vi "Main.vi"() -> ()   [LabVIEW 2021]
uses:
  Controls/Tab Control.ctl
  Controls/case control.ctl
  Controls/status_amc_entries.ctl
  Controls/assign_amc_status.ctl
  Controls/Enum.ctl
  Controls/MySQL Credential Control.ctl
panel:
  in  "error in (no error) 2":errorcluster
  in  "error in (no error)":errorcluster
  in  "Tab Control":T1
  in  "Password":string
  in  "Username":string
  in  "Login Button":bool
  in  "Role  2":T2
  in  "Assign AMC":bool
  in  "Manage Clients":bool
  in  "Report Button":bool
  in  "ADD/EDIT AMC":bool
  in  "ADD USER":bool
  in  "View All AMC":bool
  in  "Log out":bool
  in  "login Back 1":bool
  in  "Log Service Visit":bool
  in  "View Assigned AMC":bool
  in  "Update AMC":bool
  in  "login Back  2":bool
  in  "View Clients":bool
  in  "View Assign AMC":bool
  in  "View AMC":bool
  in  "Save":bool
  in  "Back":bool
  in  "Role":enum16{"admin", "engineer", "user"}(ring)
  in  "Add Username":string
  in  "Add Password":string
  in  "Delete":bool
  in  "Back Button 2":bool
  in  "User Assigned":string
  in  "Maintenance Cycle":enum16{"Quaterly", "Half Yearly", "Yearly"}(ring)
  in  "AMC Status":T3
  in  "Expiry Date":timestamp format="%<%Y/%m/%d>T"
  in  "Purchase Date":timestamp format="%<%Y/%m/%d>T"
  in  "Vendor":string
  in  "Machine":string
  in  "ADD AMC":bool
  in  "Refresh Button":bool
  in  "Back Button":bool
  out "data":string[][](table)
  in  "Back Button 4":bool
  in  "Assign":bool
  in  "Remarks":string
  in  "Status":T4
  in  "vendor":string
  in  "maintenance_cycle":string
  in  "machine_name":string
  in  "Location":string
  in  "assigned_engineer_id":dbl
  in  "engineer_remarks":string
  out "Table 3":string[][](table)
  in  "Back Button 3":bool
  in  "Back Button 5":bool
  out "Table 2":string[][](table)
  in  "Back Button 6":bool
  in  "Upload Button":bool
  in  "id 3":dbl
  in  "engineer_remarks 3":string
  in  "Back Button 7":bool
  in  "User Back Button":bool
  out "data 3":string[][](table)
  in  "User Back Button 2":bool
  out "Table":string[][](table)
  in  "User Back Button 1":bool
  out "Table 5":string[][](table)
  out "error out":errorcluster
  # "AMC TRACKER"
  # "Admin Dashboard"
  # "Engineer Dashboard"
  # "Status"
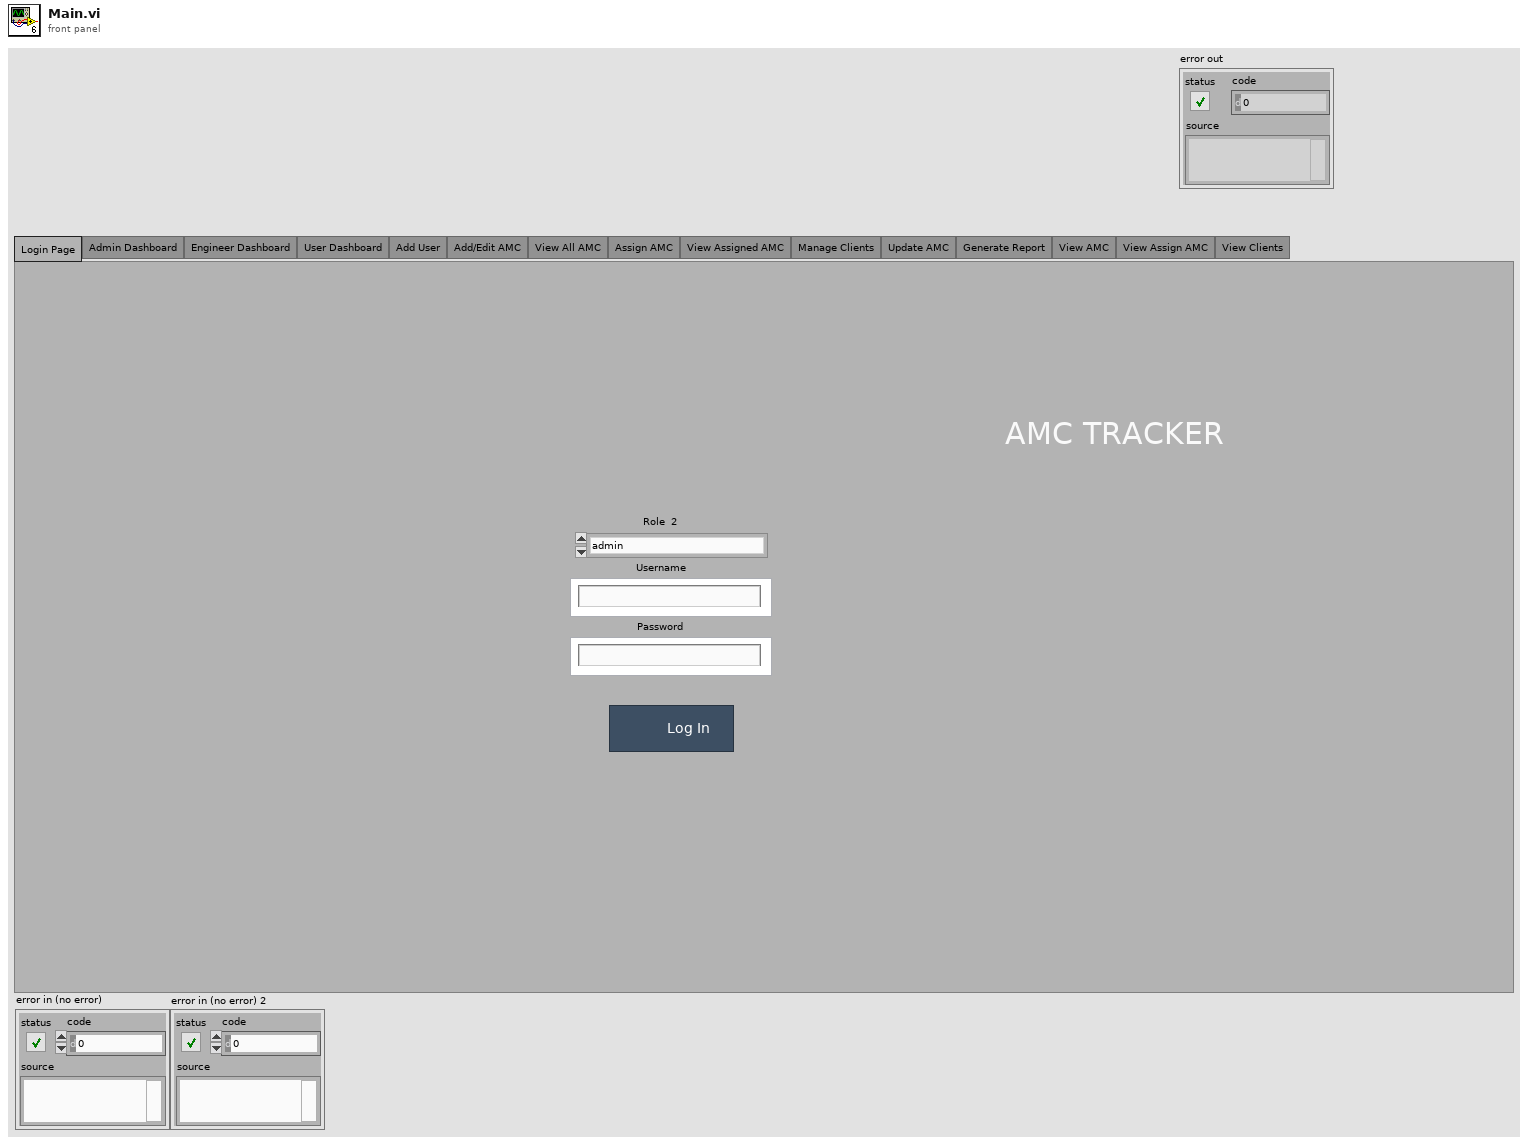
[diagram p1: front panel]
types:
  T1 = typedef "Tab Control.ctl" = enum32{"Login Page", "Admin Dashboard", "Engineer Dashboard", "User Dashboard", "Add User", "Add/Edit AMC", "View All AMC", "Assign AMC", "View Assigned AMC", "Manage Clients", "Update AMC", "Generate Report", "View AMC", "View Assign AMC", "View Clients"}
  T2 = typedef "case control.ctl" = enum16{"admin", "engineer", "user"}
  T3 = typedef "status_amc_entries.ctl" = enum16{"Active", "Expired"}
  T4 = typedef "assign_amc_status.ctl" = enum16{"Active", "Completed", "Pending"}
  T5 = typedef "Enum.ctl" = enum16{"init", "Execute Query", "Close"}
  T6 = typedef "MySQL Credential Control.ctl" = cluster{"Server":string, " User ID":string, "Password":string}
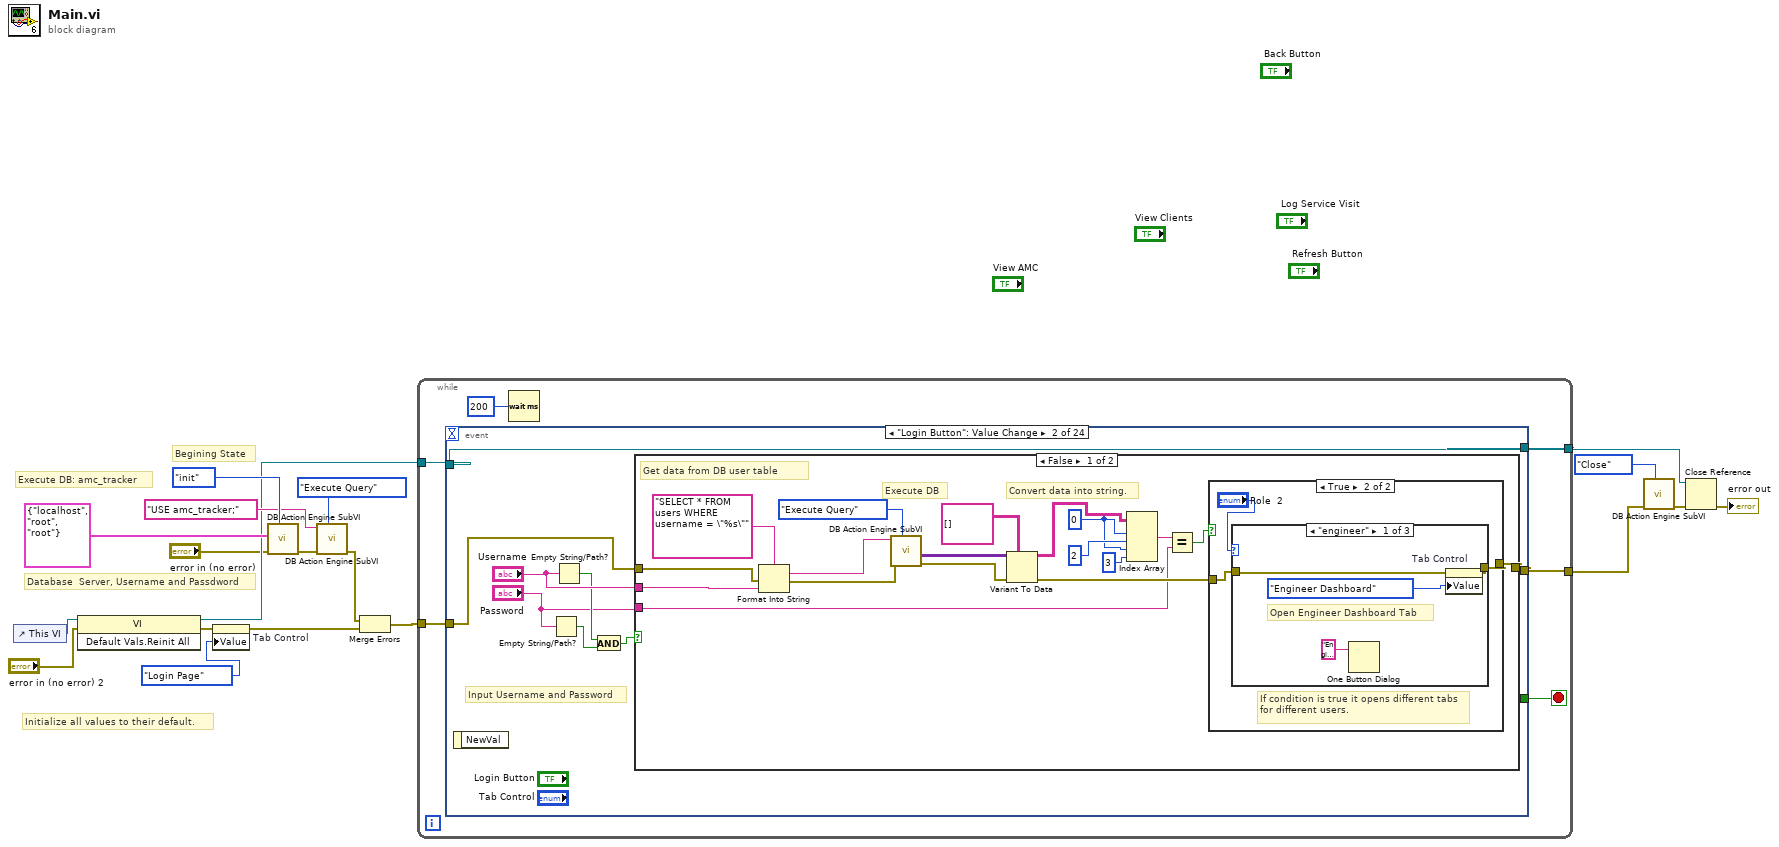
[diagram p0: block diagram]
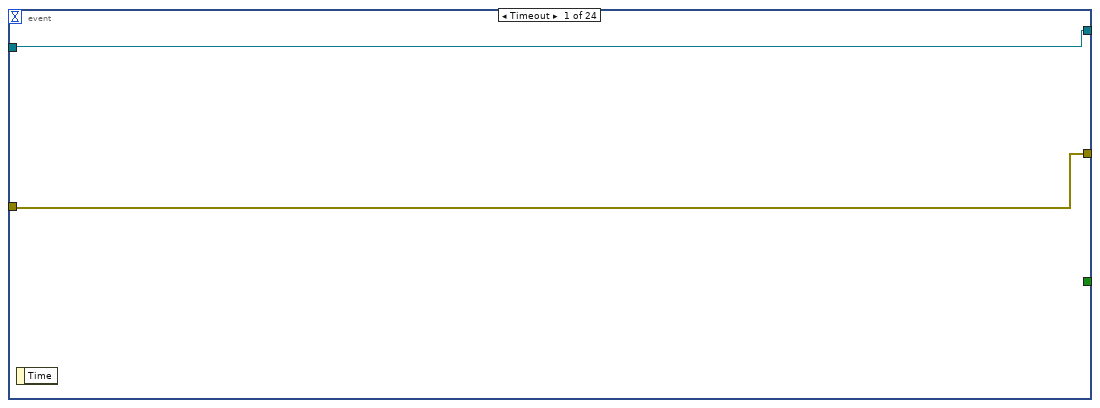
[diagram p2: hidden frame]
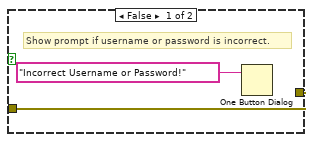
[diagram p3: hidden frame]
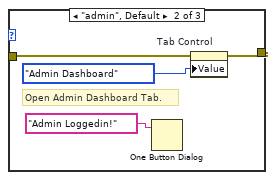
[diagram p4: hidden frame]
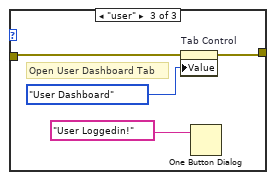
[diagram p5: hidden frame]
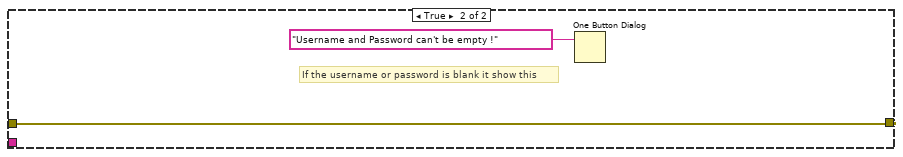
[diagram p6: hidden frame]
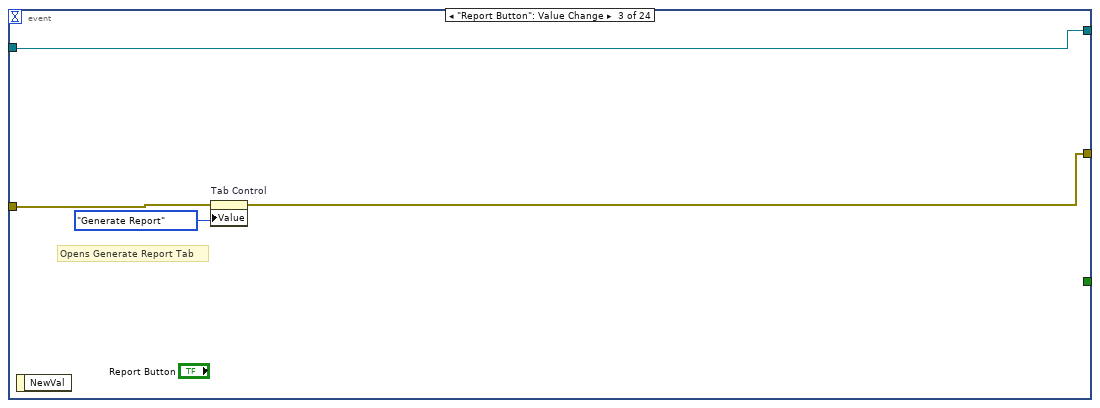
[diagram p7: hidden frame]
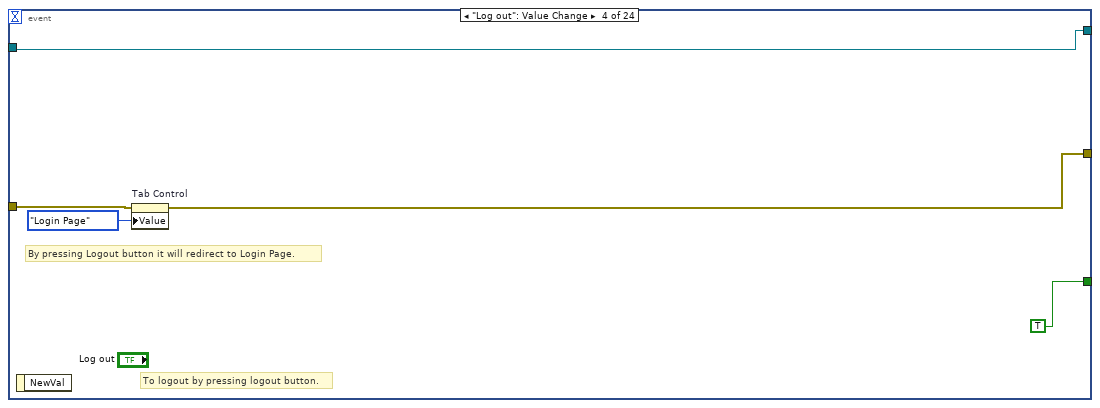
[diagram p8: hidden frame]
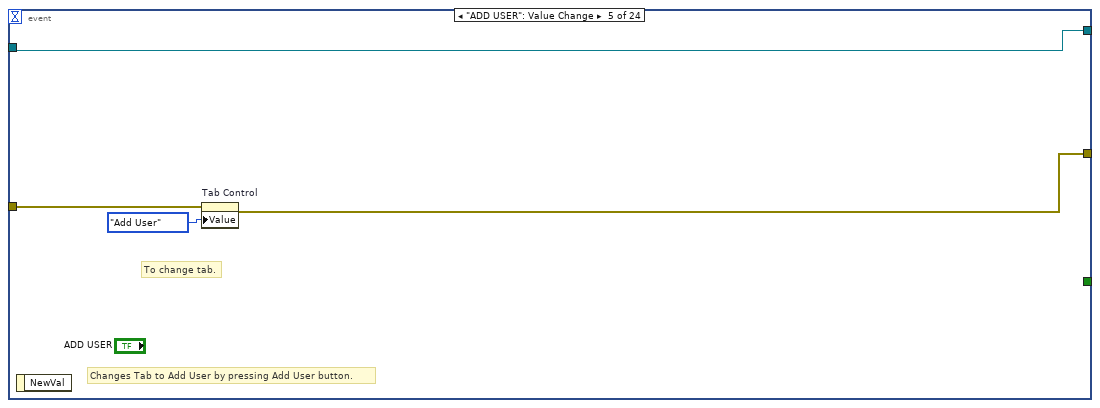
[diagram p9: hidden frame]
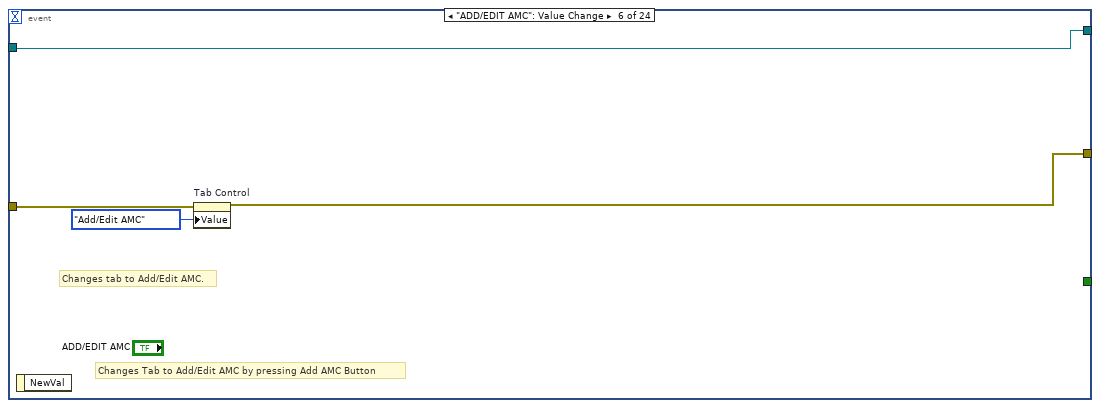
[diagram p10: hidden frame]
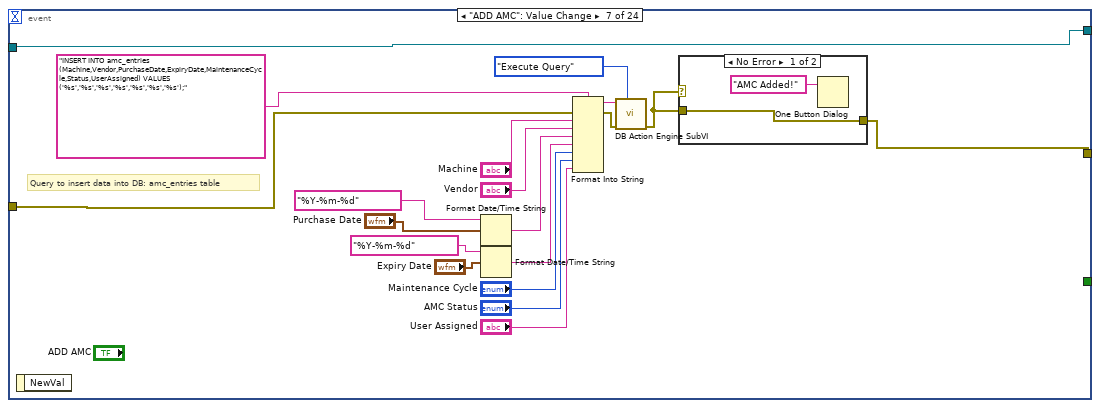
[diagram p11: hidden frame]
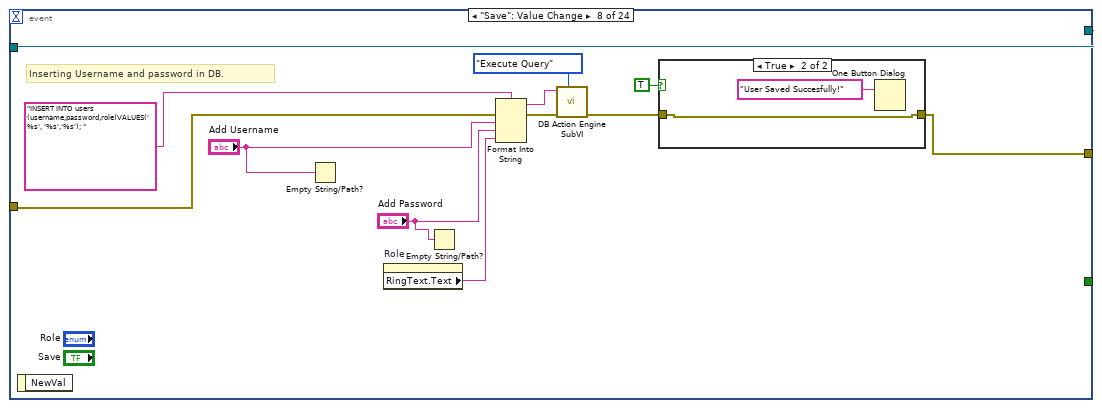
[diagram p13: hidden frame]
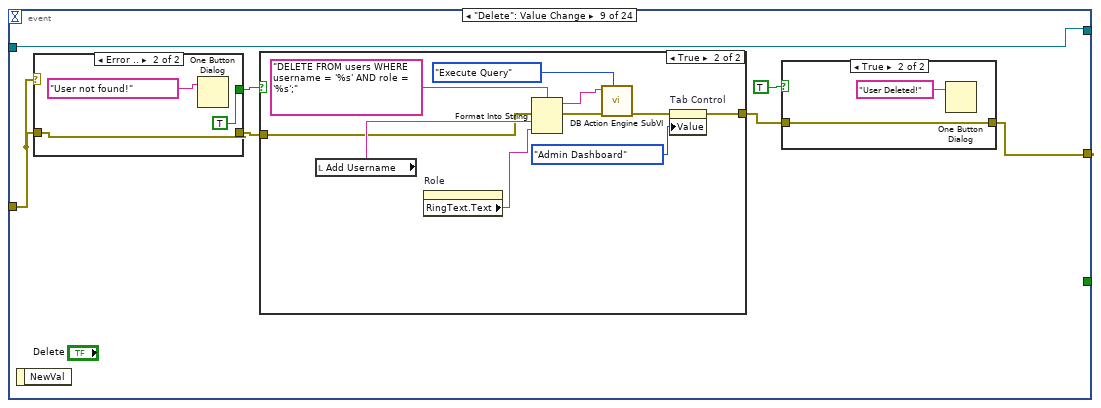
[diagram p15: hidden frame]
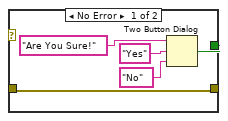
[diagram p18: hidden frame]
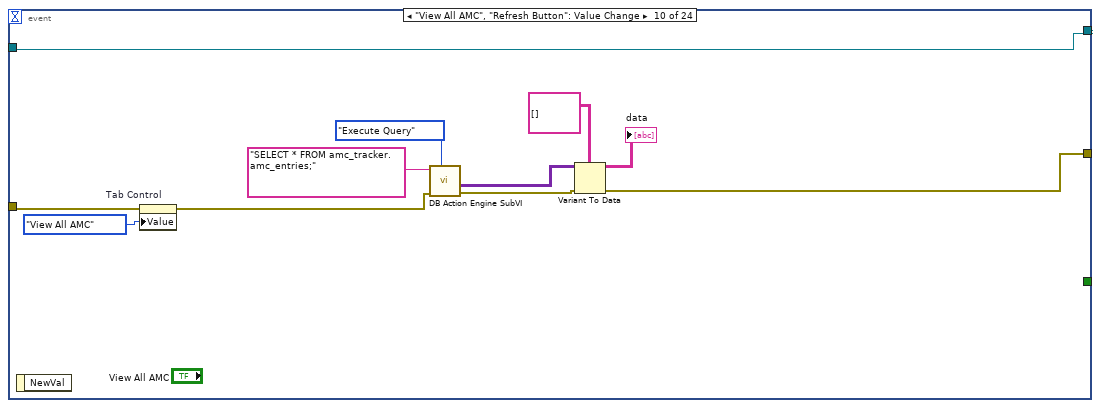
[diagram p19: hidden frame]
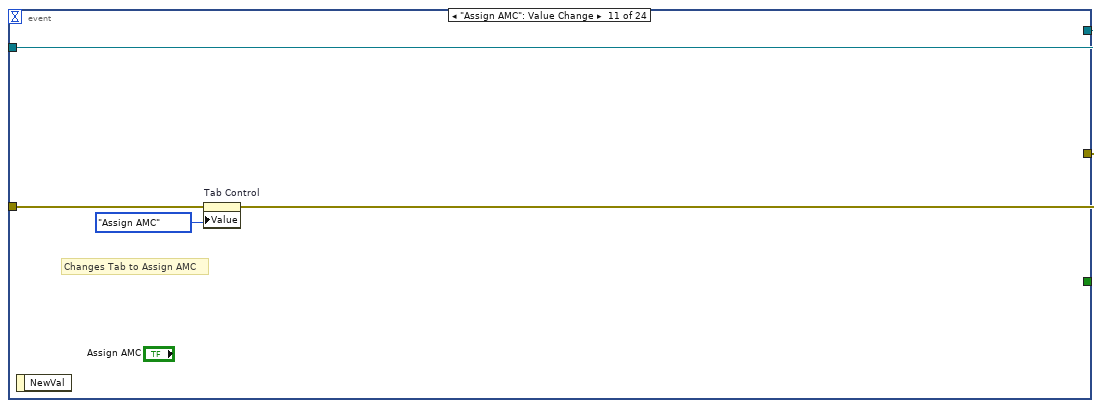
[diagram p20: hidden frame]
diagram:
  # "Database  Server, Username and Passdword"
  # "Initialize all values to their default."
  # "Execute DB: amc_tracker"
  # "Begining State"
  n1 = control-ref of="This VI"() -> (w11:refnum<vi>)
  n2 = invoke class="VI" method="Default Vals.Reinit All"(reference=w11, error in="error in (no error) 2") -> (reference out=w9:refnum<vi>, error out=w10:errorcluster)  [unwired: 1 in, 1 out]
  n3 = property on="Tab Control" class="TabCtl (strict)"(error in=w10, "Value"=Tab_Control."Login Page" ("Tab Control")) -> (error out=w3:errorcluster)  [unwired: 1 in, 1 out]
  n4 = call "DB Action Engine SubVI.vi"("Cmd"=Enum."init", "error in (no error)"="error in (no error)", "MySQL Credentials"=T6 {"Server"="localhost", " User ID"="root", "Password"="root"}) -> ("error out"=w17:errorcluster)  [unwired: 6 in, 2 out]
  n5 = call "DB Action Engine SubVI.vi"("Cmd"=Enum."Execute Query", "error in (no error)"=w17, "Query String"="USE amc_tracker;") -> ("error out"=w4:errorcluster)  [unwired: 6 in, 2 out]
  n6 = Merge Errors(w4, w3) -> (w5:errorcluster)
  n7 = while {
    tunnel: w5 -> [w25]
    tunnel: [w24] -> w14
    tunnel: w9 -> [w22]
    tunnel: [w21] -> w7
    stop <- w20 stop-if-true
    n8 = event shown="[1] \"Login Button\": Value Change" {
      selector: _ -> [_ _ _ _ _ _ _ _ _ _ _ _ _ _ _ _ _ _ _ _ _ _ _ _]
      dyn-events: _ -> [_ _ _ _ _ _ _ _ _ _ _ _ _ _ _ _ _ _ _ _ _ _ _ _]
      timeout: _ -> [_ _ _ _ _ _ _ _ _ _ _ _ _ _ _ _ _ _ _ _ _ _ _ _]
      tunnel: [_ _ _ TRUE _ _ _ _ _ _ _ _ _ _ _ _ _ _ _ _ _ _ _ _] -> w20
      tunnel: w25 -> [w27 w28 w75 w80 w83 w88 w108 w120 w127 w165 w169 w184 w188 w192 w203 w207 w210 w222 w226 w236 w255 w266 w270 w274]
      tunnel: [w27 w35 w74 w79 w84 w87 w91 w116 w129 w160 w168 w185 w187 w191 w199 w206 w213 w221 w225 w238 w247 w258 w269 w273] -> w24
      tunnel: w22 -> [w26 w29 w73 w78 w82 w86 w90 w115 w128 w156 w167 w171 w186 w190 w194 w205 w209 w220 w224 w235 w254 w265 w268 w272]
      tunnel: [w26 w29 w73 w78 w82 w86 w90 w115 w128 w156 w167 w171 w186 w190 w194 w205 w209 w220 w224 w235 w254 w265 w268 w272] -> w21
      event Timeout {
        n9 = event-data() -> ()  [unwired: 1 in, 1 out]
      }
      event "Login Button": Value Change {
        # "Input Username and Password"
        n10 = event-data() -> ()  [unwired: 1 in, 1 out]
        n11 = Empty String/Path?(string/path="Password") -> (empty?=w30:bool)
        n12 = Empty String/Path?(string/path="Username") -> (empty?=w33:bool)
        n13 = And(x=w33, y=w30) -> (x .and. y?=w31:bool)
        n14 = case shown="False" w31 {
          tunnel: w28 -> [w51 w71]
          tunnel: [w40 w71] -> w35
          tunnel: "Password" -> [w37 _]
          tunnel: "Username" -> [w36 _]
          frame False {
            w43 = 0 ("index (row)")
            # "Convert data into string."
            # "Execute DB"
            # "Get data from DB user table"
            n15 = Format Into String(format string="SELECT * FROM users WHERE username = \"%s\"" ("Query String"), error in=w51, w36) -> (resulting string=w47:string, error out=w46:errorcluster)  [unwired: 1 in]
            n16 = call "DB Action Engine SubVI.vi"("Cmd"=Enum."Execute Query", "error in (no error)"=w46, "Query String"=w47) -> ("error out"=w44:errorcluster, "data"=w39:variant[][])  [unwired: 6 in, 1 out]
            n17 = Variant To Data(error in=w44, type=string[][] [], Variant=w39) -> (data=w50:string[][], error out=w41:errorcluster)
            n18 = Index Array(array=w50, index (row) #1=w43, index (col) #1=2 ("disabled index (col)"), index (row) #2=w43, index (col) #2=3 ("disabled index (col)")) -> (element #1=w48:string)  [unwired: 1 out]
            n19 = Equal?(x=w48, y=w37) -> (x = y?=w38:bool)
            n20 = case shown="True" w38 {
              tunnel: w41 -> [w55 w58]
              tunnel: [w55 w57] -> w40
              frame False {
                # "Show prompt if username or password is incorrect."
                n21 = One Button Dialog(message="Incorrect Username or Password!") -> ()  [unwired: 1 in, 1 out]
              }
              frame True {
                # "If condition is true it opens different tabs for different users."
                n22 = case shown="\"engineer\"" "Role  2" {
                  tunnel: w58 -> [w62 w65 w70]
                  tunnel: [w61 w64 w69] -> w57
                  frame "engineer" {
                    # "Open Engineer Dashboard Tab"
                    n23 = One Button Dialog(message="Engineer Loggedin!") -> ()  [unwired: 1 in, 1 out]
                    n24 = property on="Tab Control" class="TabCtl (strict)"(error in=w62, "Value"=Tab_Control."Engineer Dashboard" ("Tab Control")) -> (error out=w61:errorcluster)  [unwired: 1 in, 1 out]
                  }
                  frame "admin", Default {
                    # "Open Admin Dashboard Tab."
                    n25 = One Button Dialog(message="Admin Loggedin!") -> ()  [unwired: 1 in, 1 out]
                    n26 = property on="Tab Control" class="TabCtl (strict)"(error in=w65, "Value"=Tab_Control."Admin Dashboard" ("Tab Control")) -> (error out=w64:errorcluster)  [unwired: 1 in, 1 out]
                  }
                  frame "user" {
                    # "Open User Dashboard Tab"
                    n27 = property on="Tab Control" class="TabCtl (strict)"(error in=w70, "Value"=Tab_Control."User Dashboard" ("Tab Control")) -> (error out=w69:errorcluster)  [unwired: 1 in, 1 out]
                    n28 = One Button Dialog(message="User Loggedin!") -> ()  [unwired: 1 in, 1 out]
                  }
                }
              }
            }
          }
          frame True {
            # "If the username or password is blank it show this"
            n29 = One Button Dialog(message="Username and Password can't be empty !") -> ()  [unwired: 1 in, 1 out]
          }
        }
      }
      event "Report Button": Value Change {
        # "Opens Generate Report Tab"
        n30 = event-data() -> ()  [unwired: 1 in, 1 out]
        n31 = property on="Tab Control" class="TabCtl (strict)"(error in=w75, "Value"=Tab_Control."Generate Report" ("Tab Control")) -> (error out=w74:errorcluster)  [unwired: 1 in, 1 out]
      }
      event "Log out": Value Change {
        # "By pressing Logout button it will redirect to Login Page."
        # "To logout by pressing logout button."
        n32 = event-data() -> ()  [unwired: 1 in, 1 out]
        n33 = property on="Tab Control" class="TabCtl (strict)"(error in=w80, "Value"=Tab_Control."Login Page" ("Tab Control")) -> (error out=w79:errorcluster)  [unwired: 1 in, 1 out]
      }
      event "ADD USER": Value Change {
        # "To change tab."
        # "Changes Tab to Add User by pressing Add User button."
        n34 = event-data() -> ()  [unwired: 1 in, 1 out]
        n35 = property on="Tab Control" class="TabCtl (strict)"(error in=w83, "Value"=Tab_Control."Add User" ("Tab Control")) -> (error out=w84:errorcluster)  [unwired: 1 in, 1 out]
      }
      event "ADD/EDIT AMC": Value Change {
        # "Changes tab to Add/Edit AMC."
        # "Changes Tab to Add/Edit AMC by pressing Add AMC Button"
        n36 = event-data() -> ()  [unwired: 1 in, 1 out]
        n37 = property on="Tab Control" class="TabCtl (strict)"(error in=w88, "Value"=Tab_Control."Add/Edit AMC" ("Tab Control")) -> (error out=w87:errorcluster)  [unwired: 1 in, 1 out]
      }
      event "ADD AMC": Value Change {
        # "Query to insert data into DB: amc_entries table"
        n38 = event-data() -> ()  [unwired: 1 in, 1 out]
        n39 = Format Date/Time String(time format string (%c)="%Y-%m-%d", seconds (now)="Purchase Date") -> (date/time string=w94:string)  [unwired: 1 in]
        n40 = Format Date/Time String(time format string (%c)="%Y-%m-%d", seconds (now)="Expiry Date") -> (date/time string=w93:string)  [unwired: 1 in]
        n41 = Format Into String(format string="INSERT INTO amc_entries (Machine,Vendor,PurchaseDate,ExpiryDate,MaintenanceCycle,Status,UserAssigned) VALUES ('%s','%s','%s','%s','%s','%s','%s');" ("Query String"), error in=w108, "Machine", "Vendor", w94, w93, "Maintenance Cycle", "AMC Status", "User Assigned") -> (resulting string=w99:string, error out=w101:errorcluster)  [unwired: 1 in]
        n42 = call "DB Action Engine SubVI.vi"("Cmd"=Enum."Execute Query", "error in (no error)"=w101, "Query String"=w99) -> ("error out"=w92:errorcluster)  [unwired: 6 in, 2 out]
        n43 = case shown="No Error" w92 {
          tunnel: w92 -> [w110 w111]
          tunnel: [w110 w111] -> w91
          frame No Error {
            n44 = One Button Dialog(message="AMC Added!") -> ()  [unwired: 1 in, 1 out]
          }
          frame Error {
          }
        }
      }
      event "Save": Value Change {
        # "Inserting Username and password in DB."
        n45 = event-data() -> ()  [unwired: 1 in, 1 out]
        n46 = Empty String/Path?(string/path="Add Username") -> ()  [unwired: 1 out]
        n47 = property on="Role" class="Enum (strict)"() -> ("RingText.Text"=w118:string)  [unwired: 2 in, 2 out]
        n48 = Empty String/Path?(string/path="Add Password") -> ()  [unwired: 1 out]
        n49 = Format Into String(format string="INSERT INTO users (username,password,role)VALUES('%s', '%s','%s'); " ("Query String"), error in=w120, "Add Username", "Add Password", w118) -> (resulting string=w121:string, error out=w122:errorcluster)  [unwired: 1 in]
        n50 = call "DB Action Engine SubVI.vi"("Cmd"=Enum."Execute Query", "error in (no error)"=w122, "Query String"=w121) -> ("error out"=w117:errorcluster)  [unwired: 6 in, 2 out]
        n51 = case shown="True" TRUE {
          tunnel: [w124 w126] -> w116
          tunnel: w117 -> [w124 w126]
          frame False {
          }
          frame True {
            n52 = One Button Dialog(message="User Saved Succesfully!") -> ()  [unwired: 1 in, 1 out]
          }
        }
      }
      event "Delete": Value Change {
        n53 = event-data() -> ()  [unwired: 1 in, 1 out]
        n54 = case shown="Error .." w127 {
          tunnel: w127 -> [w152 w155]
          tunnel: [w152 w155] -> w133
          tunnel: [w150 TRUE ("true")] -> w132
          frame No Error {
            n55 = Two Button Dialog(message="Are You Sure!", 1:"No" ("F button name (\"Cancel\")"), 2:"Yes" ("T button name (\"OK\")")) -> (T button?=w150:bool)
          }
          frame Error {
            n56 = One Button Dialog(message="User not found!") -> ()  [unwired: 1 in, 1 out]
          }
        }
        n57 = case shown="True" w132 {
          tunnel: w133 -> [w137 w138]
          tunnel: [w137 w147] -> w130
          frame False {
          }
          frame True {
            n58 = local read "Add Username"() -> (w144:string)
            n59 = property on="Role" class="Enum (strict)"() -> ("RingText.Text"=w145:string)  [unwired: 2 in, 2 out]
            n60 = Format Into String(format string="DELETE FROM users WHERE username = '%s' AND role = '%s';" ("Query String"), error in=w138, w144, w145) -> (resulting string=w143:string, error out=w142:errorcluster)  [unwired: 1 in]
            n61 = call "DB Action Engine SubVI.vi"("Cmd"=Enum."Execute Query", "error in (no error)"=w142, "Query String"=w143) -> ("error out"=w139:errorcluster)  [unwired: 6 in, 2 out]
            n62 = property on="Tab Control" class="TabCtl (strict)"(error in=w139, "Value"=Tab_Control."Admin Dashboard" ("Tab Control")) -> (error out=w147:errorcluster)  [unwired: 1 in, 1 out]
          }
        }
        n63 = case shown="True" TRUE {
          tunnel: w130 -> [w134 w136]
          tunnel: [w134 w136] -> w129
          frame False {
          }
          frame True {
            n64 = One Button Dialog(message="User Deleted!") -> ()  [unwired: 1 in, 1 out]
          }
        }
      }
      event "View All AMC", "Refresh Button": Value Change {
        n65 = event-data() -> ()  [unwired: 1 in, 1 out]
        n66 = property on="Tab Control" class="TabCtl (strict)"(error in=w165, "Value"=Tab_Control."View All AMC" ("Tab Control")) -> (error out=w164:errorcluster)  [unwired: 1 in, 1 out]
        n67 = call "DB Action Engine SubVI.vi"("Cmd"=Enum."Execute Query", "error in (no error)"=w164, "Query String"="SELECT * FROM amc_tracker.amc_entries;") -> ("error out"=w163:errorcluster, "data"=w159:variant[][])  [unwired: 6 in, 1 out]
        n68 = Variant To Data(error in=w163, type=string[][] [] ("data"), Variant=w159) -> (data=→"data":string[][], error out=w160:errorcluster)
      }
      event "Assign AMC": Value Change {
        # "Changes Tab to Assign AMC"
        n69 = event-data() -> ()  [unwired: 1 in, 1 out]
        n70 = property on="Tab Control" class="TabCtl (strict)"(error in=w169, "Value"=Tab_Control."Assign AMC" ("Tab Control")) -> (error out=w168:errorcluster)  [unwired: 1 in, 1 out]
      }
      event "Assign": Value Change {
        # "To insert data into assign_amc"
        n71 = event-data() -> ()  [unwired: 1 in, 1 out]
        n72 = Format Into String(format string="INSERT INTO assign_amc (machine_name,location,vendor,maintenance_cycle,status,assigned_engineer_id,admin_remarks,engineer_remarks) VALUES ('%s','%s','%s','%s','%s','%d','%s','%s');", error in=w184, "machine_name", "Location", "vendor", "maintenance_cycle", "Status", "assigned_engineer_id", "Remarks", "engineer_remarks") -> (resulting string=w173:string, error out=w183:errorcluster)  [unwired: 1 in]
        n73 = call "DB Action Engine SubVI.vi"("Cmd"=Enum."Execute Query", "error in (no error)"=w183, "Query String"=w173) -> ("error out"=w185:errorcluster)  [unwired: 6 in, 2 out]
      }
      event "Back Button", "Back Button 2", "Back", "Back Button 4", "Back Button 5", "Back Button 7": Value Change {
        # "Changes tab to Admin Dashboard by pressing back button"
        n74 = event-data() -> ()  [unwired: 1 in, 1 out]
        n75 = property on="Tab Control" class="TabCtl (strict)"(error in=w188, "Value"=Tab_Control."Admin Dashboard" ("Tab Control")) -> (error out=w187:errorcluster)  [unwired: 1 in, 1 out]
      }
      event "Back Button 6": Value Change {
        n76 = event-data() -> ()  [unwired: 1 in, 1 out]
        n77 = property on="Tab Control" class="TabCtl (strict)"(error in=w192, "Value"=Tab_Control."Engineer Dashboard" ("Tab Control")) -> (error out=w191:errorcluster)  [unwired: 1 in, 1 out]
      }
      event "View Assigned AMC": Value Change {
        # "Query to opens assign_amc table from amc_tracker."
        # "Changes tab to View Assigned AMC"
        n78 = event-data() -> ()  [unwired: 1 in, 1 out]
        n79 = property on="Tab Control" class="TabCtl (strict)"(error in=w203, "Value"=Tab_Control."View Assigned AMC" ("Tab Control")) -> (error out=w202:errorcluster)  [unwired: 1 in, 1 out]
        n80 = call "DB Action Engine SubVI.vi"("Cmd"=Enum."Execute Query", "error in (no error)"=w202, "Query String"="SELECT * FROM amc_tracker.assign_amc;") -> ("error out"=w200:errorcluster, "data"=w198:variant[][])  [unwired: 6 in, 1 out]
        n81 = Variant To Data(error in=w200, type=string[][] [], Variant=w198) -> (data=→"Table 3":string[][], error out=w199:errorcluster)
      }
      event "Back Button 3": Value Change {
        # "Change tab to Engineer Dashboard."
        n82 = event-data() -> ()  [unwired: 1 in, 1 out]
        n83 = property on="Tab Control" class="TabCtl (strict)"(error in=w207, "Value"=Tab_Control."Engineer Dashboard" ("Tab Control")) -> (error out=w206:errorcluster)  [unwired: 1 in, 1 out]
      }
      event "Manage Clients": Value Change {
        # "Query to show amc_clients table from amc_tracker DB."
        n84 = event-data() -> ()  [unwired: 1 in, 1 out]
        n85 = property on="Tab Control" class="TabCtl (strict)"(error in=w210, "Value"=Tab_Control."Manage Clients" ("Tab Control")) -> (error out=w218:errorcluster)  [unwired: 1 in, 1 out]
        n86 = call "DB Action Engine SubVI.vi"("Cmd"=Enum."Execute Query", "error in (no error)"=w218, "Query String"="SELECT * FROM amc_tracker.amc_clients;") -> ("error out"=w215:errorcluster, "data"=w214:variant[][])  [unwired: 6 in, 1 out]
        n87 = Variant To Data(error in=w215, type=string[][] [], Variant=w214) -> (data=→"Table 2":string[][], error out=w213:errorcluster)
      }
      event "Update AMC": Value Change {
        # "Changes tab to Update AMC by pressing Update AMC Button."
        n88 = event-data() -> ()  [unwired: 1 in, 1 out]
        n89 = property on="Tab Control" class="TabCtl (strict)"(error in=w222, "Value"=Tab_Control."Update AMC" ("Tab Control")) -> (error out=w221:errorcluster)  [unwired: 1 in, 1 out]
      }
      event "Upload Button": Value Change {
        # "Upload engineer remarks to assign table"
        n90 = event-data() -> ()  [unwired: 1 in, 1 out]
        n91 = property on="Tab Control" class="TabCtl (strict)"(error in=w226, "Value"=Tab_Control."Update AMC" ("Tab Control")) -> (error out=w232:errorcluster)  [unwired: 1 in, 1 out]
        n92 = Format Into String(initial string="UPDATE assign_amc SET engineer_remarks = '%s' WHERE id = '%d';", error in=w232, "engineer_remarks 3", "id 3") -> (resulting string=w230:string, error out=w231:errorcluster)  [unwired: 1 in]
        n93 = call "DB Action Engine SubVI.vi"("Cmd"=Enum."Execute Query", "error in (no error)"=w231, "Query String"=w230) -> ("error out"=w225:errorcluster)  [unwired: 6 in, 2 out]
      }
      event "View AMC": Value Change {
        n94 = event-data() -> ()  [unwired: 1 in, 1 out]
        n95 = property on="Tab Control" class="TabCtl (strict)"(error in=w236, "Value"=Tab_Control."View AMC" ("Tab Control")) -> (error out=w239:errorcluster)  [unwired: 1 in, 1 out]
        n96 = call "DB Action Engine SubVI.vi"("Cmd"=Enum."Execute Query", "error in (no error)"=w239, "Query String"="SELECT * FROM amc_tracker.amc_entries;") -> ("error out"=w242:errorcluster, "data"=w241:variant[][])  [unwired: 6 in, 1 out]
        n97 = Variant To Data(error in=w242, type=string[][] [], Variant=w241) -> (data=→"data 3":string[][], error out=w238:errorcluster)
      }
      event "View Assign AMC": Value Change {
        n98 = event-data() -> ()  [unwired: 1 in, 1 out]
        n99 = property on="Tab Control" class="TabCtl (strict)"(error in=w255, "Value"=Tab_Control."View Assign AMC" ("Tab Control")) -> (error out=w248:errorcluster)  [unwired: 1 in, 1 out]
        n100 = call "DB Action Engine SubVI.vi"("Cmd"=Enum."Execute Query", "error in (no error)"=w248, "Query String"="SELECT * FROM amc_tracker.assign_amc;") -> ("error out"=w251:errorcluster, "data"=w250:variant[][])  [unwired: 6 in, 1 out]
        n101 = Variant To Data(error in=w251, type=string[][] [], Variant=w250) -> (data=→"Table 5":string[][], error out=w247:errorcluster)
      }
      event "View Clients": Value Change {
        n102 = event-data() -> ()  [unwired: 1 in, 1 out]
        n103 = property on="Tab Control" class="TabCtl (strict)"(error in=w266, "Value"=Tab_Control."View Clients" ("Tab Control")) -> (error out=w259:errorcluster)  [unwired: 1 in, 1 out]
        n104 = call "DB Action Engine SubVI.vi"("Cmd"=Enum."Execute Query", "error in (no error)"=w259, "Query String"="SELECT * FROM amc_tracker.amc_clients;") -> ("error out"=w264:errorcluster, "data"=w263:variant[][])  [unwired: 6 in, 1 out]
        n105 = Variant To Data(error in=w264, type=string[][] [], Variant=w263) -> (data=→"Table":string[][], error out=w258:errorcluster)
      }
      event "User Back Button", "User Back Button 1", "User Back Button 2": Value Change {
        n106 = event-data() -> ()  [unwired: 1 in, 1 out]
        n107 = property on="Tab Control" class="TabCtl (strict)"(error in=w270, "Value"=Tab_Control."User Dashboard" ("Tab Control")) -> (error out=w269:errorcluster)  [unwired: 1 in, 1 out]
      }
      event "login Back 1", "login Back  2": Value Change {
        n108 = event-data() -> ()  [unwired: 1 in, 1 out]
        n109 = property on="Tab Control" class="TabCtl (strict)"(error in=w274, "Value"=Tab_Control."Login Page" ("Tab Control")) -> (error out=w273:errorcluster)  [unwired: 1 in, 1 out]
      }
    }
    n110 = Wait (ms)(milliseconds to wait=u32 200) -> ()  [unwired: 1 out]
  }
  n111 = call "DB Action Engine SubVI.vi"("Cmd"=Enum."Close", "error in (no error)"=w14) -> ("error out"=w8:errorcluster)  [unwired: 7 in, 2 out]
  n112 = Close Reference(reference=w7, error in (no error)=w8) -> (error out=→"error out":errorcluster)
